vi "Read Key Names.vi"(8 "error in":errorcluster, 11 "Config in":refnum<class "Config.lvclass">) -> (0 "error out":errorcluster, 3 "Config out":refnum<class "Config.lvclass">)   [LabVIEW 2023, in "Config.lvlib" / "Config.lvclass"]
uses:
  Config.lvclass
  Config.lvclass/Config.ctl
  <vilib>/Utility/config.llb/NI_LVConfig.lvlib
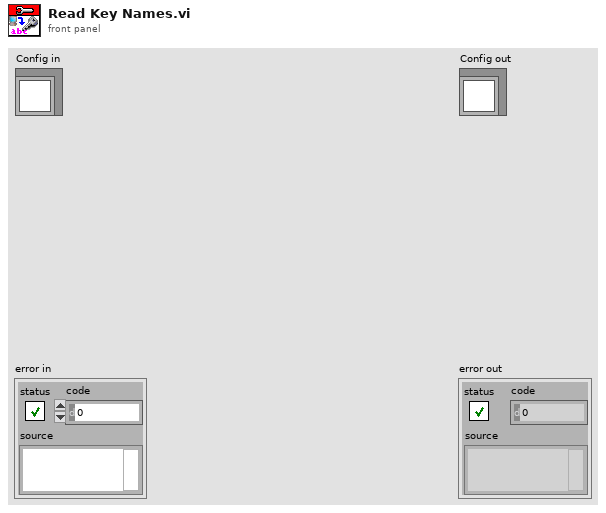
[diagram p1: front panel]
types:
  T1 = typedef "NI_LVConfig.lvlib/Config Data RefNum.ctl" = refnum<k1>
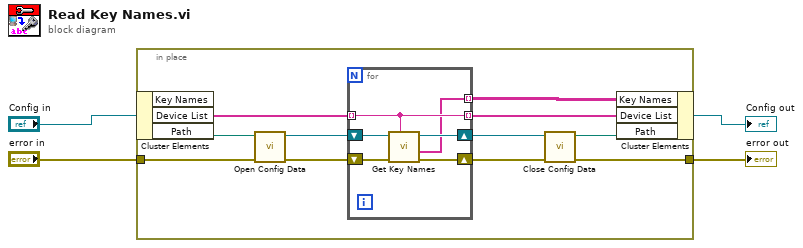
[diagram p0: block diagram]
diagram:
  n1 = in-place {
    in-place-border: "error in" -> [w9]
    in-place-border: [w8] -> w1
    n2 = in-place-cluster #1("Config in") -> ("Device List"=w7:string[], "Path"=w15:path)  [unwired: 1 out]
    n3 = call <vilib>:"Open Config Data.vi"("error in (no error)"=w9, "configuration file path"=w15) -> ("error out"=w13:errorcluster, "refnum"=w14:T1)  [unwired: 7 in, 1 out]
    n4 = for {
      shift-right: [w19] -> w12
      shift-left: w14 -> [w21]
      shift-right: [w18] -> w11
      shift-left: w13 -> [w20]
      tunnel: w7 -> [w17] mode=indexing
      tunnel: [w17] -> w6 mode=indexing
      tunnel: [w16] -> w5 mode=indexing
      n5 = call <vilib>:"Get Key Names.vi"("section"=w17, "error in (no error)"=w20, "refnum"=w21) -> ("error out"=w18:errorcluster, "key names"=w16:string[], "refnum out"=w19:T1)  [unwired: 5 in, 1 out]
    }
    n6 = call <vilib>:"Close Config Data.vi"("error in (no error)"=w11, "refnum"=w12) -> ("error out"=w8:errorcluster, "file path"=w10:path)  [unwired: 8 in]
    n7 = in-place-cluster #1("Key Names"=w5, "Device List"=w6, "Path"=w10) -> (→"Config out":refnum<class "Config.lvclass">)
  }
  "error out" <- w1
